vi "Calculate Flow Rate.vi"(7 "GCF data source (Bronkhorst)":u16(ring) items=["Bronkhorst", "Brooks", "MKS"], 8 "error in (no error)":errorcluster, 9 "actual gas/mixture":string(combo)="Ar", 10 "calibration gas":string(combo)="N2", 11 "measured gas flow rate":dbl) -> (0 "error out":errorcluster, 3 "actual gas flow rate":dbl)   [LabVIEW 2015, in "PL GCF Calculator.lvlib"]
doc: "Calculates <b>actual gas flow rate</b> based on <b>measured gas flow rate</b>, mfc <b>calibration gas</b>, <b>actual gas/mixture</b> and <b>GCF data source</b>.\nMixture string example: \"80% Ar + 20% O2\"."
uses:
  PL GCF Calculator.lvlib
  <vilib>/Utility/file.llb/Read Delimited Spreadsheet (string).vi
panel:
  out "gases":string[](array[string])
  out "GCFs":dbl[](array[numeric])
  out "current GCF data source":u16(ring) items=["Bronkhorst", "Brooks", "MKS"]
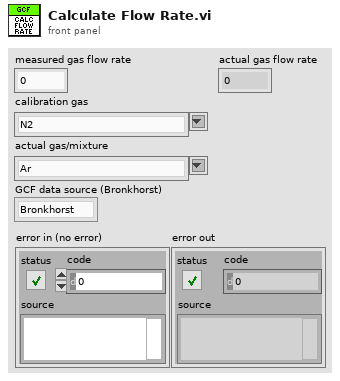
[diagram p1: front panel]
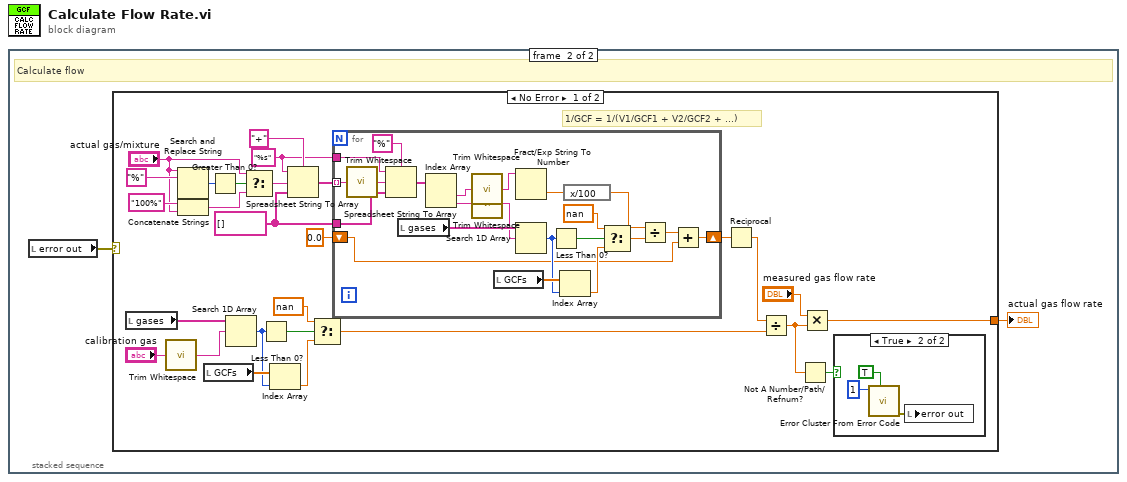
[diagram p0: block diagram]
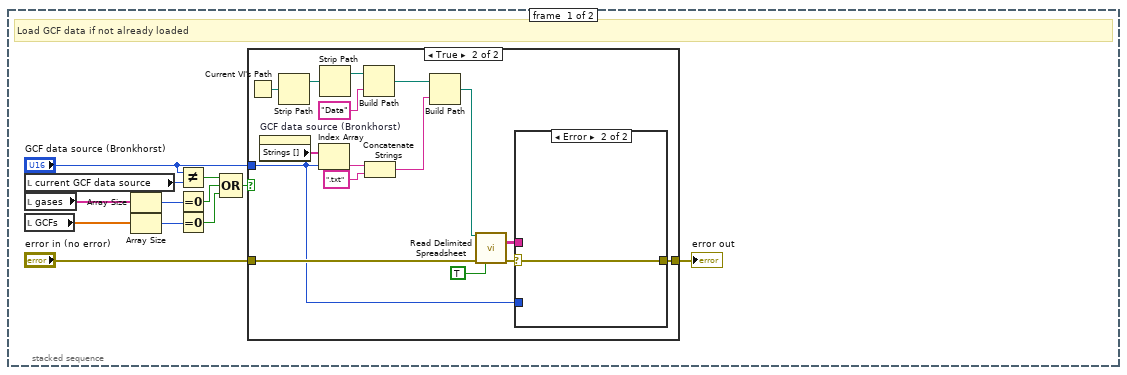
[diagram p2: hidden frame]
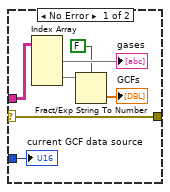
[diagram p4: hidden frame]
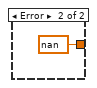
[diagram p6: hidden frame]
diagram:
  n1 = stacked-sequence {
    frame #0 {
      # "Load GCF data if not already loaded"
      n2 = local read "current GCF data source"() -> (w12:u16)
      n3 = local read "gases"() -> (w10:string[])
      n4 = local read "GCFs"() -> (w3:dbl[])
      n5 = Array Size(array=w10) -> (size(s)=w9:i32)
      n6 = Array Size(array=w3) -> (size(s)=w2:i32)
      n7 = Not Equal?(x="GCF data source (Bronkhorst)", y=w12) -> (x != y?=w11:bool)
      n8 = Equal To 0?(x=w9) -> (x = 0?=w8:bool)
      n9 = Equal To 0?(x=w2) -> (x = 0?=w1:bool)
      n10 = Compound Arithmetic op=OR(w11, w8, w1) -> (w7:bool)
      n11 = case shown="True" w7 {
        tunnel: "GCF data source (Bronkhorst)" -> [_ w16]
        tunnel: "error in (no error)" -> [w13 w20]
        tunnel: [w13 w17] -> w4
        frame False {
        }
        frame True {
          n12 = Current VI's Path() -> (path=w24:path)
          n13 = property on="GCF data source (Bronkhorst)" class="Ring (strict)"() -> ("Strings []"=w29:string[])  [unwired: 2 in, 2 out]
          n14 = Strip Path(path=w24) -> (stripped path=w15:path)  [unwired: 1 out]
          n15 = Index Array(array=w29, index=w16) -> (element=w28:string)
          n16 = Strip Path(path=w15) -> (stripped path=w14:path)  [unwired: 1 out]
          n17 = Build Path(base path=w14, name or relative path="Data") -> (appended path=w26:path)
          n18 = Concatenate Strings(w28, ".txt" ("string")) -> (w23:string)
          n19 = Build Path(base path=w26, name or relative path=w23) -> (appended path=w22:path)
          n20 = call-poly <vilib>:"Read Delimited Spreadsheet.vi"("file path (dialog if empty)"=w22, "error in (no error)"=w20, "transpose? (F)"=TRUE) -> ("all rows"=w19:string[][], "error out"=w18:errorcluster)  [unwired: 7 in, 4 out]
          n21 = case shown="Error" w18 {
            selector: w18 -> [w35 w37]
            tunnel: w19 -> [w36 _]
            tunnel: [w35 w37] -> w17
            tunnel: w16 -> [w34 _]
            frame No Error {
              n22 = Index Array(array=w36) -> (element #1=→"gases":string[], element #2=w31:string[])  [unwired: 4 in]
              n23 = Fract/Exp String To Number(use system decimal point (T)=FALSE, string=w31) -> (number=→"GCFs":dbl[])  [unwired: 2 in, 1 out]
              "current GCF data source" <- w34
            }
            frame Error {
            }
          }
        }
      }
      "error out" <- w4
    }
    frame #1 {
      # "Calculate flow"
      n24 = local read "error out"() -> (w39:errorcluster)
      n25 = case shown="No Error" w39 {
        tunnel: [w41 nan] -> w38
        frame No Error {
          w56 = "%s" ("format string")
          w57 = string[] [] ("array type (2D Dbl)")
          # "1/GCF = 1/(V1/GCF1 + V2/GCF2 + ...)"
          n26 = local read "gases"() -> (w48:string[])
          n27 = call <vilib>:"Trim Whitespace.vi"("string"="calibration gas") -> ("trimmed string"=w40:string)  [unwired: 1 in]
          n28 = Search and Replace String(input string="actual gas/mixture", search string="%") -> (number of replacements=w65:i32)  [unwired: 6 in, 3 out]
          n29 = Concatenate Strings("100%" ("string"), "actual gas/mixture") -> (w61:string)
          n30 = local read "GCFs"() -> (w53:dbl[])
          n31 = Greater Than 0?(x=w65) -> (x > 0?=w64:bool)
          n32 = Search 1D Array(1D array=w48, element=w40) -> (index of element=w52:i32)  [unwired: 1 in]
          n33 = Select(t="actual gas/mixture", s=w64, f=w61) -> (s? t:f=w59:string)
          n34 = Less Than 0?(x=w52) -> (x < 0?=w50:bool)
          n35 = Index Array(array=w53, index=w52) -> (element=w51:dbl)
          n36 = Spreadsheet String To Array(delimiter (Tab)="+", format string=w56, spreadsheet string=w59, array type (2D Dbl)=w57) -> (array=w58:string[])
          n37 = Select(t=nan, s=w50, f=w51) -> (s? t:f=w45:dbl)
          n38 = for {
            tunnel: w58 -> [w91] mode=indexing
            tunnel: w57 -> [w90]
            tunnel: w56 -> [w71]
            shift-right: [w73] -> w54
            shift-left: 0.0 -> [w72]
            n39 = call <vilib>:"Trim Whitespace.vi"("string"=w91) -> ("trimmed string"=w70:string)  [unwired: 1 in]
            n40 = Spreadsheet String To Array(delimiter (Tab)="%", format string=w71, spreadsheet string=w70, array type (2D Dbl)=w90) -> (array=w88:string[])
            n41 = local read "gases"() -> (w84:string[])
            n42 = Index Array(array=w88) -> (element #1=w86:string, element #2=w87:string)  [unwired: 2 in]
            n43 = call <vilib>:"Trim Whitespace.vi"("string"=w86) -> ("trimmed string"=w85:string)  [unwired: 1 in]
            n44 = call <vilib>:"Trim Whitespace.vi"("string"=w87) -> ("trimmed string"=w83:string)  [unwired: 1 in]
            n45 = local read "GCFs"() -> (w82:dbl[])
            n46 = Fract/Exp String To Number(string=w85) -> (number=w77:dbl)  [unwired: 3 in, 1 out]
            n47 = Search 1D Array(1D array=w84, element=w83) -> (index of element=w81:i32)  [unwired: 1 in]
            n48 = Less Than 0?(x=w81) -> (x < 0?=w79:bool)
            n49 = Index Array(array=w82, index=w81) -> (element=w80:dbl)
            n50 = expression code="x/100"(w77) -> (w76:dbl)
            n51 = Select(t=nan, s=w79, f=w80) -> (s? t:f=w75:dbl)
            n52 = Divide(x=w76, y=w75) -> (x/y=w74:dbl)
            n53 = Add(x=w74, y=w72) -> (x+y=w73:dbl)
          }
          n54 = Reciprocal(x=w54) -> (1/x=w46:dbl)
          n55 = Divide(x=w46, y=w45) -> (x/y=w43:dbl)
          n56 = Not A Number/Path/Refnum?(number/path/refnum=w43) -> (NaN/Path/Refnum?=w42:bool)
          n57 = Multiply(x="measured gas flow rate", y=w43) -> (x*y=w41:dbl)
          n58 = case shown="True" w42 {
            frame False {
            }
            frame True {
              n59 = call <vilib>:"Error Cluster From Error Code.vi"("show call chain? (False)"=TRUE, "error code (0)"=1) -> ("error out"=w67:errorcluster)  [unwired: 7 in]
              n60 = local write "error out"(w67) -> ()
            }
          }
        }
        frame Error {
        }
      }
      "actual gas flow rate" <- w38
    }
  }
